vi "Cluster Experiment.vi"() -> ()   [LabVIEW 2014]
panel:
  out "Small Cluster":cluster{"Boolean 1":bool, "Slide Value":dbl}
  out "Modified Cluster":T1 {"Slide" scale=0.0..10.0}
  in  "Cluster":T1 {"Slide" scale=0.0..10.0}
  out "Boolean 2":bool
  out "Numeric":dbl
  in  "stop":bool
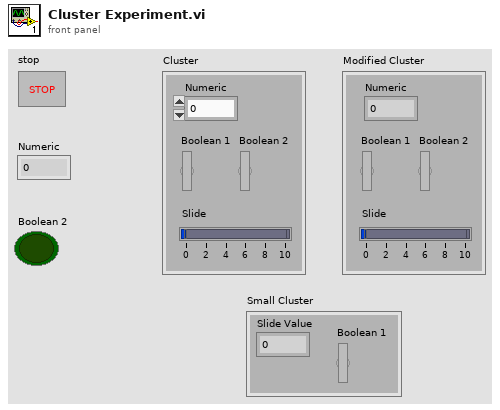
[diagram p1: front panel]
types:
  T1 = cluster{"Numeric":dbl, "Boolean 1":bool, "Boolean 2":bool, "Slide":dbl}
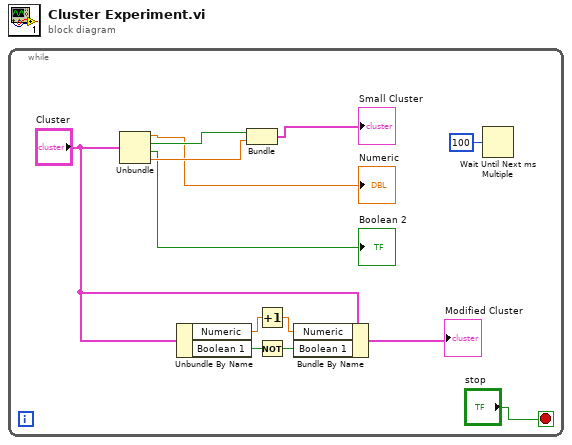
[diagram p0: block diagram]
diagram:
  n1 = while {
    stop <- "stop" stop-if-true
    n2 = Unbundle("Cluster") -> ("Numeric"=→"Numeric":dbl, "Boolean 1"=w12:bool, "Boolean 2"=→"Boolean 2":bool, "Slide"=w11:dbl)
    n3 = Unbundle By Name("Cluster") -> ("Numeric"=w9:dbl, "Boolean 1"=w7:bool)
    n4 = Bundle("Boolean 1"=w12, "Slide"=w11) -> (→"Small Cluster":cluster{"Boolean 1":bool, "Slide":dbl})  [unwired: 1 in]
    n5 = Increment(x=w9) -> (x+1=w8:dbl)
    n6 = Not(x=w7) -> (.not. x?=w4:bool)
    n7 = Bundle By Name(cluster="Cluster", "Numeric"=w8, "Boolean 1"=w4) -> (→"Modified Cluster":T1)
    n8 = Wait Until Next ms Multiple(millisecond multiple=u32 100) -> ()  [unwired: 1 out]
  }
